vi "find tagetdata.vi"(9 "target":enum16{"主舱外回路", "主舱内回路", "实验舱外回路", "实验舱内回路"}(ring), 10 "CalData":T2(array[cluster])) -> (1 "data":T1, 2 "find?":bool)   [LabVIEW 2011]
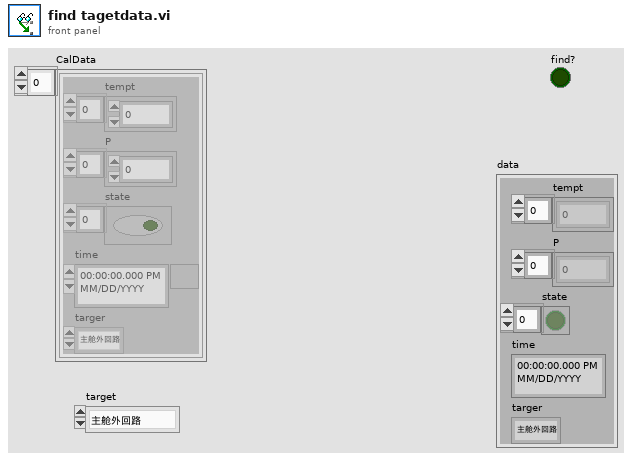
[diagram p1: front panel]
types:
  T1 = cluster{"tempt":dbl[], "P":dbl[], "state":bool[], "time":timestamp, "targer":enum16{"主舱外回路", "主舱内回路", "实验舱外回路", "实验舱内回路"}}
  T2 = cluster{"tempt":dbl[], "P":dbl[], "state":bool[], "time":timestamp, "targer":enum16{"主舱外回路", "主舱内回路", "实验舱外回路", "实验舱内回路"}}[]
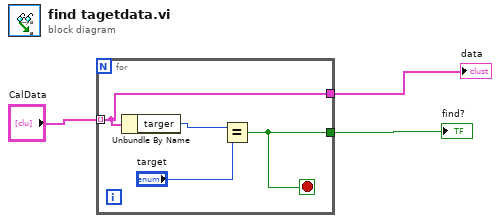
[diagram p0: block diagram]
diagram:
  n1 = for {
    tunnel: "CalData" -> [w5] mode=indexing
    tunnel: [w4] -> w2
    tunnel: [w5] -> w1
    stop <- w4 stop-if-true
    n2 = Unbundle By Name(w5) -> ("targer"=w7:enum16{"主舱外回路", "主舱内回路", "实验舱外回路", "实验舱内回路"})
    n3 = Equal?(x=w7, y="target") -> (x = y?=w4:bool)
  }
  "find?" <- w2
  "data" <- w1
